vi "HowdyDrive.vi"(6 "HighGear?":bool, 8 "error in (no error)":errorcluster, 9 "Y":dbl, 10 "X":dbl, 11 "Pod Drive in":refnum<class "Pod Drive.lvclass">) -> (0 "error out":errorcluster, 3 "Pod Drive out":refnum<class "Pod Drive.lvclass">)   [LabVIEW 2018, in "Drive.lvlib" / "Pod Drive.lvclass"]
doc: "Runs motors based of joystick values in velocity closed loop mode, a version of arcade drive with support for CTRE motor controllers"
uses:
  Pod Drive.lvclass
  C:/Users/Public/Documents/2019DeepSpace/Classes/Drive/Drive.lvclass
  Drive.lvclass/Drive.ctl
  Pod Drive.lvclass/Pod Drive.ctl
  <vilib>/Rock Robotics/SystemInterfaces/NetworkCommunication/NetComm_UsageReport_ResourceType.ctl
  Public Methods/Read Motion Magic Constants.vi
  <vilib>/Rock Robotics/WPI/Utilities/WPI_GetSetVariantRefNum.vi
  Drive.lvclass
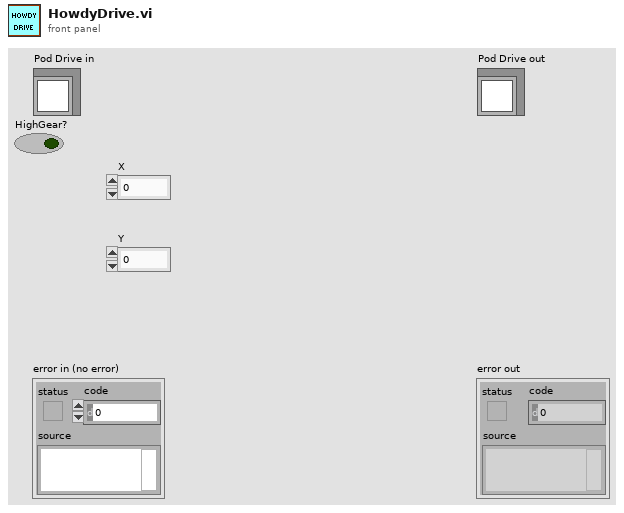
[diagram p1: front panel]
types:
  T1 = typedef "NetComm_UsageReport_ResourceType.ctl" = enum8{"Controller", "Module", "Language", "CANPlugin", "Accelerometer", "ADXL345", "AnalogChannel", "AnalogTrigger", "AnalogTriggerOutput", "CANJaguar", "Compressor", "Counter", "Dashboard", "DigitalInput", "DigitalOutput", "DriverStationCIO", "DriverStationEIO", "DriverStationLCD", "Encoder", "GearTooth", "Gyro", "I2C", "Framework", "Jaguar", "Joystick", "Kinect", "KinectStick", "PIDController", "Preferences", "PWM", "Relay", "RobotDrive", "SerialPort", "Servo", "Solenoid", "SPI", "Task", "Ultrasonic", "Victor", "Button", "Command", "AxisCamera", "PCVideoServer", "SmartDashboard", "Talon", "HiTechnicColorSensor", "HiTechnicAccel", "HiTechnicCompass", "SRF08", "AnalogOutput", "Victor SP", "Talon SRX", "CAN Talon SRX", "ADXL362 Accel", "ADXRS450 Gyro", "Rev SPARK", "Mindsensors SD540", "Digital Filter", "ADIS16448", "PDP", "PCM", "PigeonIMU", "Nidec Brushless", "CTRE CANifier", "CTRE Future 0", "CTRE Future 1", "CTRE Future 2", "CTRE Future 3", "CTRE Future 4", "CTRE Future 5", "CTRE Future 6", "Linear Filter", "Xbox Controller", "USB Camera", "NavX", "Pixy", "Pixy2", "ScanseSweep", "Shuffleboard", "CAN", "Digilent DMC60", "PWM Victor SPX", "Rev SPARK MAX PWM", "Rev SPARK MAX CAN", "ADIS16470"}
  T2 = typedef "Drive.lvlib/Drive.lvclass/Motion Magic Constants.ctl" = cluster{"Low Gear Max Velocity":u32, "High Gear Max Velocity":u32, "Motion Magic Low Gear Max Velocity":u32, "Motion Magic Low Gear Max Acceleration":u32, "Motion Magic High Gear Max Velocity":u32, "Motion Magic High Gear Max Acceleration":u32}
  T3 = typedef "WPI_RobotDriveDevRef.ctl" = cluster{"DevStatus":errorcluster, "Motors[]":T4[], "Square Inputs":bool, "Max Output":dbl}
  T4 = typedef "WPI_MotorControlDeviceRef.ctl" = cluster{"DeviceStatus":errorcluster, "Type":T5, "PWM":cluster{"PWM Channel":T6, "DeadBand":T7}, "CAN":cluster{"Device Number":u8, "SetOutput VI Ref":variant, "GetOutput VI Ref":variant, "Enable VI Ref":variant, "Disable VI Ref":variant, "Data":variant}, "Invert":bool, "DIO PWM":cluster{"PWM \"Enable\" Channel":T6, "DIOChannel":T8, "PWM Rate":dbl}}
  T5 = typedef "WPI_MotorControlType.ctl" = enum16{"PWM", "CAN", "DIO PWM"}
  T6 = typedef "FPGA_DIOPWMChannel.ctl" = enum8{"PWM 0", "PWM 1", "PWM 2", "PWM 3", "PWM 4", "PWM 5", "PWM 6", "PWM 7", "PWM 8", "PWM 9", "PWM MXP 0", "PWM MXP 1", "PWM MXP 2", "PWM MXP 3", "PWM MXP 4", "PWM MXP 5", "PWM MXP 6", "PWM MXP 7", "PWM MXP 8", "PWM MXP 9", "Invalid"}
  T7 = typedef "WPI_PWMDeadband.ctl" = cluster{"Name":string, "maxPositivePwm":i32, "minPositivePwm":i32, "centerPwm":i32, "maxNegativePwm":i32, "minNegativePwm":i32, "angularRange":u16}
  T8 = typedef "FPGA_DIOChannel.ctl" = enum8{"DIO 0", "DIO 1", "DIO 2", "DIO 3", "DIO 4", "DIO 5", "DIO 6", "DIO 7", "DIO 8", "DIO 9", "DIO MXP 0", "DIO MXP 1", "DIO MXP 2", "DIO MXP 3", "DIO MXP 4", "DIO MXP 5", "DIO MXP 6", "DIO MXP 7", "DIO MXP 8", "DIO MXP 9", "DIO MXP 10", "DIO MXP 11", "DIO MXP 12", "DIO MXP 13", "DIO MXP 14", "DIO MXP 15", "SPI Port CS1", "SPI Port CS2", "SPI Port CS3", "SPI Port MISO", "SPI Port MOSI", "Invalid"}
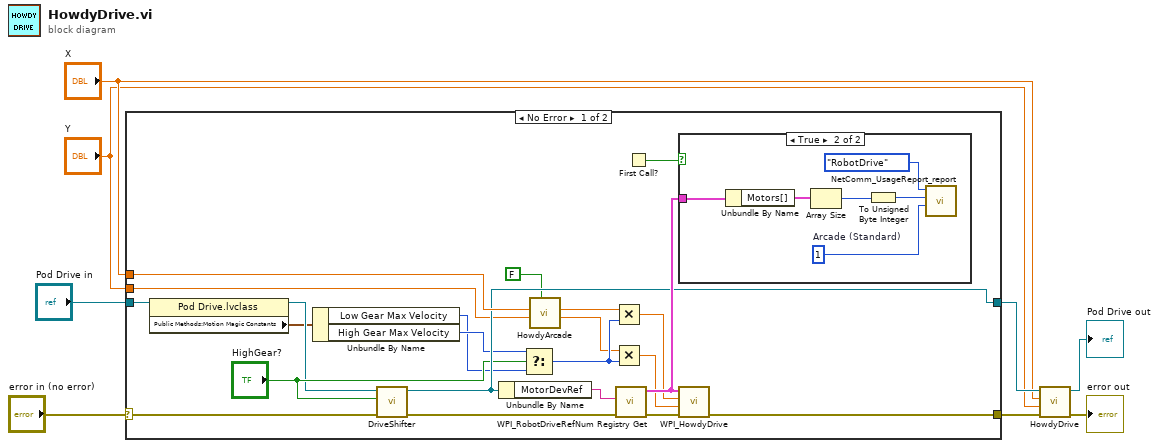
[diagram p0: block diagram]
diagram:
  n1 = case shown="No Error" "error in (no error)" {
    selector: "error in (no error)" -> [w22 w38]
    tunnel: [w20 w38] -> w2
    tunnel: [w17 w37] -> w6
    tunnel: "Pod Drive in" -> [w18 w37]
    tunnel: "X" -> [w27 _]
    tunnel: "Y" -> [w11 _]
    frame No Error {
      n2 = property class="Pod Drive.lvclass"(reference=w18) -> (reference out=w15:refnum<class "Pod Drive.lvclass">, "Public Methods:Motion Magic Constants"=w14:T2)  [unwired: 1 in, 1 out]
      n3 = Unbundle By Name(w14) -> ("Low Gear Max Velocity"=w12:u32, "High Gear Max Velocity"=w13:u32)
      n4 = call-dynamic "DriveShifter.vi"("error in (no error)"=w22, "HighGear?"="HighGear?", "Pod Drive in"=w15) -> ("error out"=w19:errorcluster, "Pod Drive out"=w17:refnum<class "Pod Drive.lvclass">)  [unwired: 7 in]
      n5 = Unbundle By Name(w17) -> ("MotorDevRef"=w29:string)
      n6 = Select(t=w13, s="HighGear?", f=w12) -> (s? t:f=w23:u32)
      n7 = call "HowdyArcade.vi"("Negate Right input (true)"=FALSE, "forward"=w11, "right"=w27) -> ("right_wheel"=w10:dbl, "left_wheel"=w25:dbl)  [unwired: 7 in]
      n8 = Multiply(x=w25, y=w23) -> (x*y=w24:dbl)
      n9 = Multiply(x=w10, y=w23) -> (x*y=w26:dbl)
      n10 = call <vilib>:"WPI_RobotDriveRefNum Registry Get.vi"("error in (no error)"=w19, "refnum name"=w29) -> ("error out"=w21:errorcluster, "RobotDriveDevRef"=w28:T3)  [unwired: 8 in]
      n11 = First Call?() -> (First Call?: T/F=w30:bool)
      n12 = case shown="True" w30 {
        tunnel: w28 -> [_ w32]
        frame False {
        }
        frame True {
          w34 = u8 1  # Arcade (Standard)
          n13 = Unbundle By Name(w32) -> ("Motors[]"=w31:T4[])
          n14 = Array Size(array=w31) -> (size(s)=w33:i32)
          n15 = To Unsigned Byte Integer(number=w33) -> (unsigned 8bit integer=w35:u8)
          n16 = call <vilib>:"NetComm_UsageReport_report.vi"("Context"=w34, "Instance Number"=w35, "Resource Type"=NetComm_UsageReport_ResourceType."RobotDrive") -> ()  [unwired: 9 in]
        }
      }
      n17 = call "WPI_HowdyDrive.vi"("error in (no error)"=w21, "RightSpeed"=w26, "LeftSpeed"=w24, "RobotDriveDevRef 2"=w28) -> ("error out"=w20:errorcluster)  [unwired: 6 in, 1 out]
    }
    frame Error {
    }
  }
  n18 = call-parent "HowdyDrive.vi"("error in (no error)"=w2, "Y"="Y", "X"="X", "Drive in"=w6) -> ("error out"=→"error out":errorcluster, "Drive out"=→"Pod Drive out":refnum<class "Pod Drive.lvclass">)  [unwired: 6 in]
